vi "Global Shutter Variables - SubVI.vi"() -> ()   [LabVIEW 2014]
uses:
  ctts/laser shutters.ctl
  ctts/user event shutter global.ctl
panel:
  in  "shutter-external-trigger":refnum<user-event>
  in  "Filterwheel Serial port":refnum<visa-resource-name>="COM1"
  in  "Laser Shutter":T1
  in  "Camera Shutter 2":bool
  out "Camera Shutter":bool[](array[boolean])
  out "Shutter In Use":string
  # "Interactive Use"
  # "***********Non-interactive Use*************"
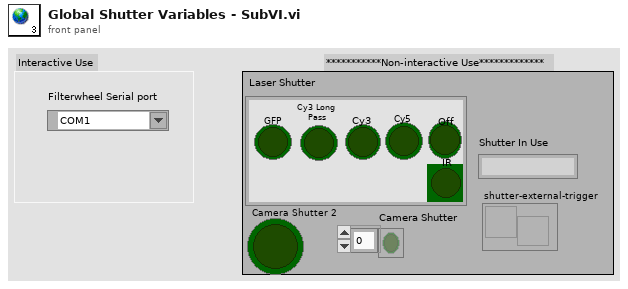
[diagram p1: front panel]
types:
  T1 = typedef "laser shutters.ctl" = enum32{"No Selection", "GFP", "Cy3 Long \nPass", "Cy3", "Cy5", "Off", "IR"}
diagram:
